vi "Stringhandling(SubVI)0.0.2.vi"(0 "Slide (Eingang)":refnum<vi>, 1 "Numerisch (Eingang)":i32, 3 "VISA-Referenz (Eingang)":refnum<visa-resource-name>, 4 "MessFrequenz [Hz]":dbl, 5 "Bytes at Port":u32, 7 "Fehler (Eingang, kein Fehler)":errorcluster, 8 "Cyclecounter (Eingang)":i32, 9 "Rolle[Hz]":dbl, 11 "Datei COM":refnum<file>, 12 "String (Eingang)":string, 13 "Zündung [Hz] (Eingang)":dbl, 15 "Datei LV-Interpretation":refnum<file>) -> (14 "Lesepuffer":string="\n", 16 "Numerisch (Ausgang)":i32, 17 "String (Ausgang)":string, 20 "VISA-Referenz (Ausgang)":refnum<visa-resource-name>, 21 "Zündung [Hz] (Ausgang)":dbl, 23 "Rolle [Hz]":dbl, 24 "Messfrequenz [Hz]":dbl, 25 "Cyclecounter (Ausgang)":i32, 27 "Fehler (Ausgang)":errorcluster)   [LabVIEW 2014]
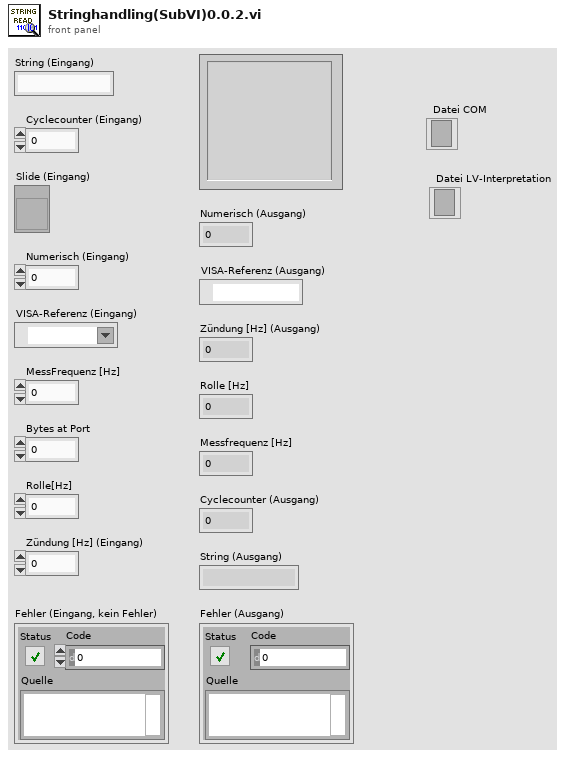
[diagram p1: front panel]
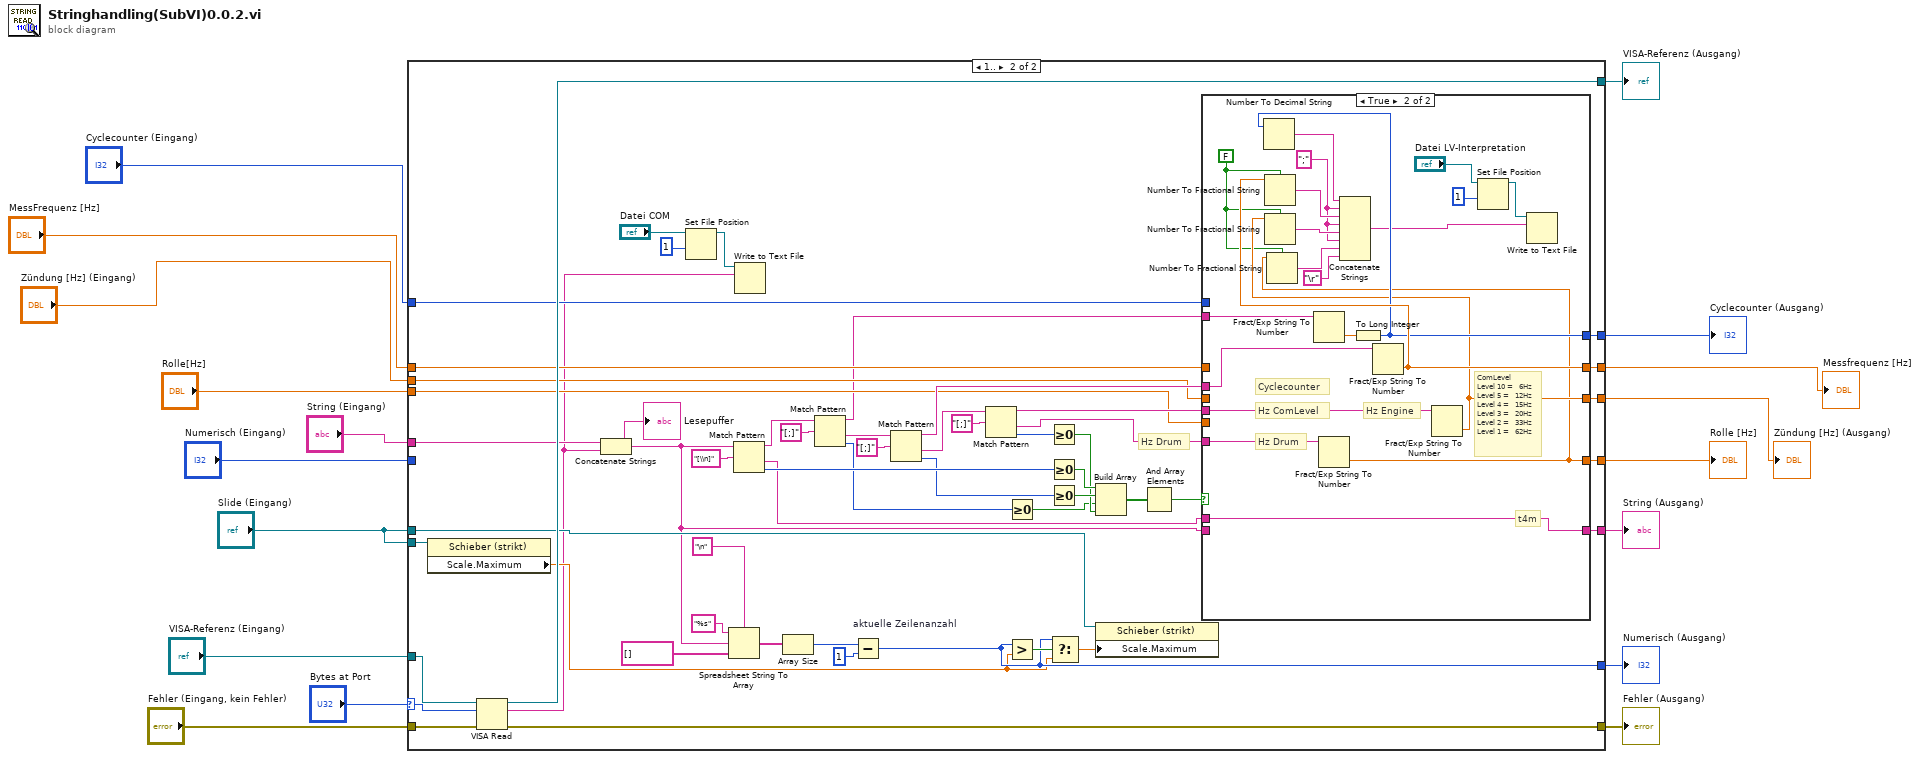
[diagram p0: block diagram]
diagram:
  n1 = case shown="1.." "Bytes at Port" {
    selector: "Bytes at Port" -> [_ w75]
    tunnel: [w20 w69] -> w10
    tunnel: [w19 w70] -> w15
    tunnel: [w24 w71] -> w8
    tunnel: [w25 w68] -> w7
    tunnel: "String (Eingang)" -> [w26 w29]
    tunnel: [w26 w66] -> w2
    tunnel: "Zündung [Hz] (Eingang)" -> [w25 w58]
    tunnel: "Rolle[Hz]" -> [w24 w57]
    tunnel: [w21 w56] -> w11
    tunnel: "MessFrequenz [Hz]" -> [w21 w55]
    tunnel: "Numerisch (Eingang)" -> [w23 _]
    tunnel: [w23 w39] -> w9
    tunnel: [w22 w44] -> w12
    tunnel: "Cyclecounter (Eingang)" -> [w22 w43]
    tunnel: "VISA-Referenz (Eingang)" -> [w19 w36]
    tunnel: "Fehler (Eingang, kein Fehler)" -> [w20 w35]
    tunnel: "Slide (Eingang)" -> [_ w34]
    tunnel: "Slide (Eingang)" -> [_ w33]
    frame 0, Default {
      # "No data in from serial port - Nothing to do."
    }
    frame 1.. {
      # "Hz Drum"
      n2 = property on="Eigenschaftsknoten" class="Schieber (strikt)"(reference=w34) -> ("Scale.Maximum"=w38:dbl)  [unwired: 1 in, 2 out]
      n3 = VISA Read(VISA resource name=w36, byte count=w75, error in (no error)=w35) -> (VISA resource name out=w70:refnum<visa-resource-name>, read buffer=w27:string, error out=w69:errorcluster)  [unwired: 1 out]
      n4 = Concatenate Strings(w29, w27) -> (w28:string)
      "Lesepuffer" <- w28
      n5 = Set File Position(refnum="Datei COM", from (0:start)=1) -> (refnum out=w30:refnum<file>)  [unwired: 2 in, 1 out]
      n6 = Spreadsheet String To Array(delimiter (Tab)="\n" ("regular expression"), format string="%s" ("regular expression"), spreadsheet string=w28, array type (2D Dbl)=string[] [] ("Array 2")) -> (array=w49:string[])
      n7 = Match Pattern(string=w28, regular expression="[\\n]") -> (before substring=w47:string, after substring=w67:string, offset past match=w79:i32)  [unwired: 1 in, 1 out]
      n8 = Write to Text File(file (use dialog)=w30, text=w27) -> ()  [unwired: 2 in, 3 out]
      n9 = Array Size(array=w49) -> (size(s)=w53:i32)
      n10 = Match Pattern(string=w47, regular expression="[;]") -> (before substring=w45:string, after substring=w46:string, offset past match=w42:i32)  [unwired: 1 in, 1 out]
      n11 = Subtract "aktuelle Zeilenanzahl"(x=w53, y=1) -> (x-y=w39:i32)
      n12 = Match Pattern(string=w46, regular expression="[;]") -> (before substring=w74:string, after substring=w77:string, offset past match=w64:i32)  [unwired: 1 in, 1 out]
      n13 = Match Pattern(string=w77, regular expression="[;]") -> (before substring=w73:string, after substring=w72:string, offset past match=w62:i32)  [unwired: 1 in, 1 out]
      n14 = Greater Or Equal To 0?(x=w42) -> (x >= 0?=w41:bool)
      n15 = Greater?(x=w39, y=w38) -> (0:w40:bool)
      n16 = Greater Or Equal To 0?(x=w62) -> (x >= 0?=w61:bool)
      n17 = Greater Or Equal To 0?(x=w79) -> (x >= 0?=w65:bool)
      n18 = Greater Or Equal To 0?(x=w64) -> (x >= 0?=w63:bool)
      n19 = Select(t=w39, s=w40, f=w38) -> (s? t:f=w37:dbl)
      n20 = Build Array(w65, w63, w41, w61) -> (w60:bool[])
      n21 = property on="Eigenschaftsknoten" class="Schieber (strikt)"(reference=w33, "Scale.Maximum"=w37) -> ()  [unwired: 1 in, 2 out]
      n22 = And Array Elements(Boolean array=w60) -> (logical AND=w59:bool)
      n23 = case shown="True" w59 {
        tunnel: w74 -> [_ w103]
        tunnel: w73 -> [_ w102]
        tunnel: w72 -> [_ w101]
        tunnel: [w83 w92] -> w71
        tunnel: [w84 w96] -> w68
        tunnel: w67 -> [_ w106]
        tunnel: [w85 w106] -> w66
        tunnel: w28 -> [w85 _]
        tunnel: w58 -> [w84 _]
        tunnel: w57 -> [w83 _]
        tunnel: [w82 w100] -> w56
        tunnel: w55 -> [w82 _]
        tunnel: w45 -> [_ w104]
        tunnel: [w81 w99] -> w44
        tunnel: w43 -> [w81 _]
        frame False {
        }
        frame True {
          w94 = ";"
          w93 = FALSE
          # "Cyclecounter"
          # "Hz ComLevel"
          # "ComLevel\nLevel 10 =   6Hz \nLevel 5 =   12Hz \nLevel 4 =   15Hz\nLevel 3 =   20Hz\nLevel 2 =   33Hz\nLevel 1 =   62Hz"
          # "Hz Drum"
          # "Hz Engine"
          # "t4m"
          n24 = Fract/Exp String To Number(string=w104) -> (number=w105:dbl)  [unwired: 3 in, 1 out]
          n25 = Fract/Exp String To Number(string=w101) -> (number=w92:dbl)  [unwired: 3 in, 1 out]
          n26 = Number To Fractional String(use system decimal point (T)=w93, number=w92) -> (F-format string=w91:string)  [unwired: 2 in]
          n27 = To Long Integer(number=w105) -> (32bit integer=w99:i32)
          n28 = Number To Decimal String(number=w99) -> (decimal integer string=w98:string)  [unwired: 1 in]
          n29 = Fract/Exp String To Number(string=w103) -> (number=w100:dbl)  [unwired: 3 in, 1 out]
          n30 = Number To Fractional String(use system decimal point (T)=w93, number=w100) -> (F-format string=w97:string)  [unwired: 2 in]
          n31 = Fract/Exp String To Number(string=w102) -> (number=w96:dbl)  [unwired: 3 in, 1 out]
          n32 = Number To Fractional String(use system decimal point (T)=w93, number=w96) -> (F-format string=w95:string)  [unwired: 2 in]
          n33 = Concatenate Strings(w98, w94, w97, w94, w95, w94, w91, "\r") -> (w90:string)
          n34 = Set File Position(refnum="Datei LV-Interpretation", from (0:start)=1) -> (refnum out=w87:refnum<file>)  [unwired: 2 in, 1 out]
          n35 = Write to Text File(file (use dialog)=w87, text=w90) -> ()  [unwired: 2 in, 3 out]
        }
      }
    }
  }
  "VISA-Referenz (Ausgang)" <- w15
  "Cyclecounter (Ausgang)" <- w12
  "Messfrequenz [Hz]" <- w11
  "Fehler (Ausgang)" <- w10
  "Numerisch (Ausgang)" <- w9
  "Rolle [Hz]" <- w8
  "Zündung [Hz] (Ausgang)" <- w7
  "String (Ausgang)" <- w2
